vi "test_find_consecutive_close_data_with_a_reference.vi"() -> ()   [LabVIEW 2024]
uses:
  <vilib>/Utility/file.llb/Read Delimited Spreadsheet (string).vi
panel:
  out "average":dbl
  in  "csv_data_ file_name":string(combo)="low-1.csv"
  in  "python_module_name":string="find_consecutive_close_values_with_a_reference.py"
  out "Measures Plot":dbl[][](graph)
  out "data qty":i32
  out "close values":dbl[](array[numeric])
  in  "tolerance%":dbl=4.0 min=0.0 format="%#.4f"
  in  "reference [W]":dbl=48.0 format="%.2f"
  # "Powered by \nPython 3.9.13\n32-bits"
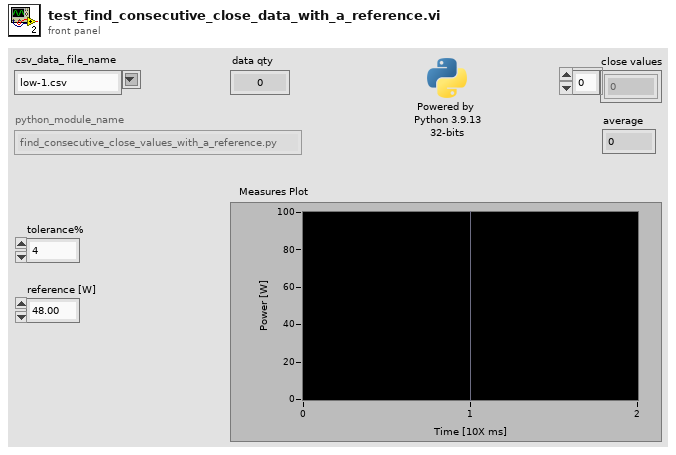
[diagram p1: front panel]
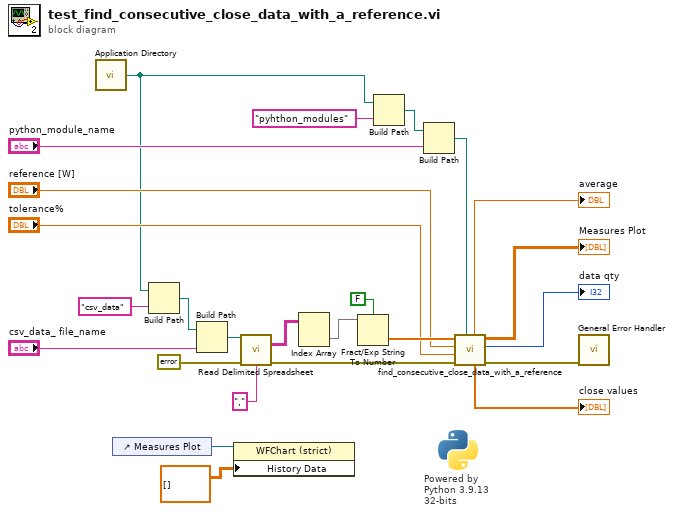
[diagram p0: block diagram]
diagram:
  # "Powered by \nPython 3.9.13\n32-bits"
  n1 = call <vilib>:"Application Directory.vi"() -> ("Application Directory"=w4:path)
  n2 = control-ref of="Measures Plot"() -> (w20:refnum<vi>)
  n3 = Build Path(base path=w4, name or relative path="csv_data") -> (appended path=w8:path)
  n4 = Build Path(base path=w8, name or relative path="csv_data_ file_name") -> (appended path=w5:path)
  n5 = property class="WFChart (strict)"(reference=w20, "History Data"=dbl[][] []) -> ()  [unwired: 1 in, 2 out]
  n6 = call-poly <vilib>:"Read Delimited Spreadsheet.vi"("file path (dialog if empty)"=w5, "error in (no error)"=errorcluster {"status"=FALSE, "code"=0, "source"=""} ("error constant"), "delimiter (\\t)"=",") -> ("all rows"=w24:string[][], "error out"=w18:errorcluster)  [unwired: 7 in, 4 out]
  n7 = Index Array(array=w24) -> (element=w22:string[])  [unwired: 2 in]
  n8 = Fract/Exp String To Number(use system decimal point (T)=FALSE, string=w22) -> (number=w16:dbl[])  [unwired: 2 in, 1 out]
  n9 = Build Path(base path=w4, name or relative path="pyhthon_modules") -> (appended path=w9:path)
  n10 = Build Path(base path=w9, name or relative path="python_module_name") -> (appended path=w3:path)
  n11 = call "find_consecutive_close_data_with_a_reference.vi"("Python module path"=w3, "error in (no error)"=w18, "Tol %"="tolerance%", "Ref [W]"="reference [W]", "data"=w16) -> ("error out"=w17:errorcluster, "data qty"=→"data qty":i32, "Measures"=→"Measures Plot":dbl[][], "close values"=→"close values":dbl[], "average"=→"average":dbl)  [unwired: 1 in, 1 out]
  n12 = call <vilib>:"General Error Handler.vi"("error in (no error)"=w17) -> ()  [unwired: 10 in, 5 out]
